vi "Plot Times.vi"(8 "reference 2":refnum<vi>, 9 "reference":refnum<vi>, 11 "Value":T1(array[cluster])) -> (0 "Positive Graph":cluster{dbl, dbl, i32[]}[](graph) caption="Waveform Graph", 3 "Negative Graph":cluster{dbl, dbl, i32[]}[](graph) caption="Waveform Graph")   [LabVIEW 2013]
doc: "Given Time Sequence Clusters, outputs vertical lines indicating relative Times\nPlots to a negative and a positive graph to allow for different scaling"
panel:
  out "Positive Graph":cluster{"X":dbl, "Y":dbl}[](graph)
  out "Negative Graph":cluster{"X":dbl, "Y":dbl}[](graph)
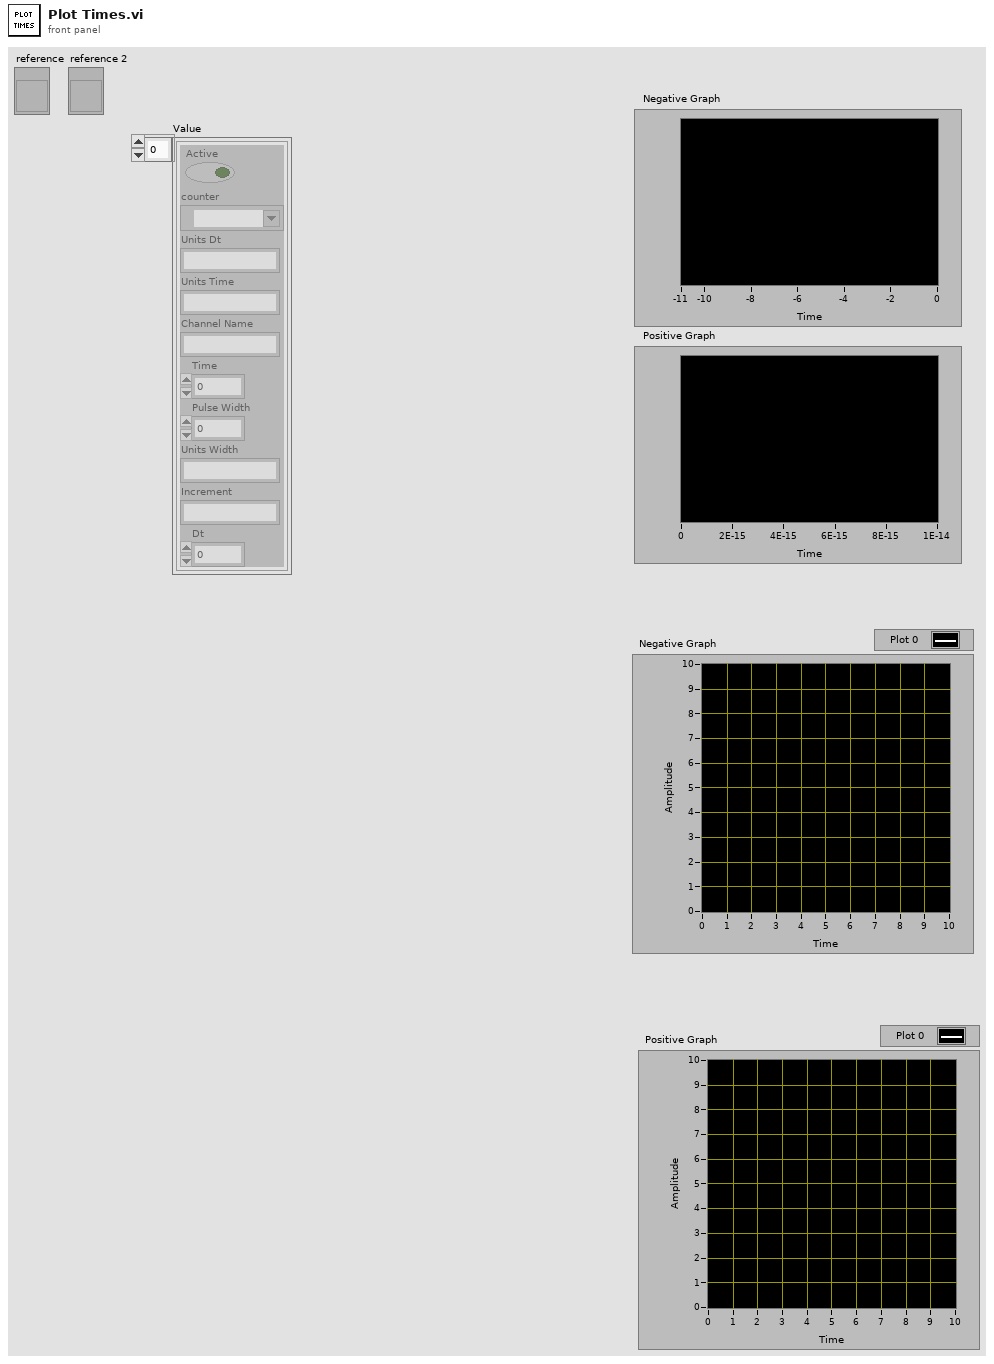
[diagram p1: front panel]
types:
  T1 = cluster{"Active":bool, "counter":tag, "Units Dt":string, "Units Time":string, "Channel Name":string, "Time":dbl, "Pulse Width":dbl, "Units Width":string, "Increment":string, "Dt":dbl}[]
  T2 = cluster{"Name":string, "Color":u32, "Style":u8, "Point Style":u8, "Name Visible":bool, "Allow Drag":bool, "Annotation Mode":u32, "Plot":i32, "Index":i32, "Position":cluster{"X":dbl, "Y":dbl}, "X Scale":u32, "Y Scale":u32, "Show Arrow":bool, "Lock Name":bool, "Plot Area":i32, "Label Offset":cluster{"X":dbl, "Y":dbl}}
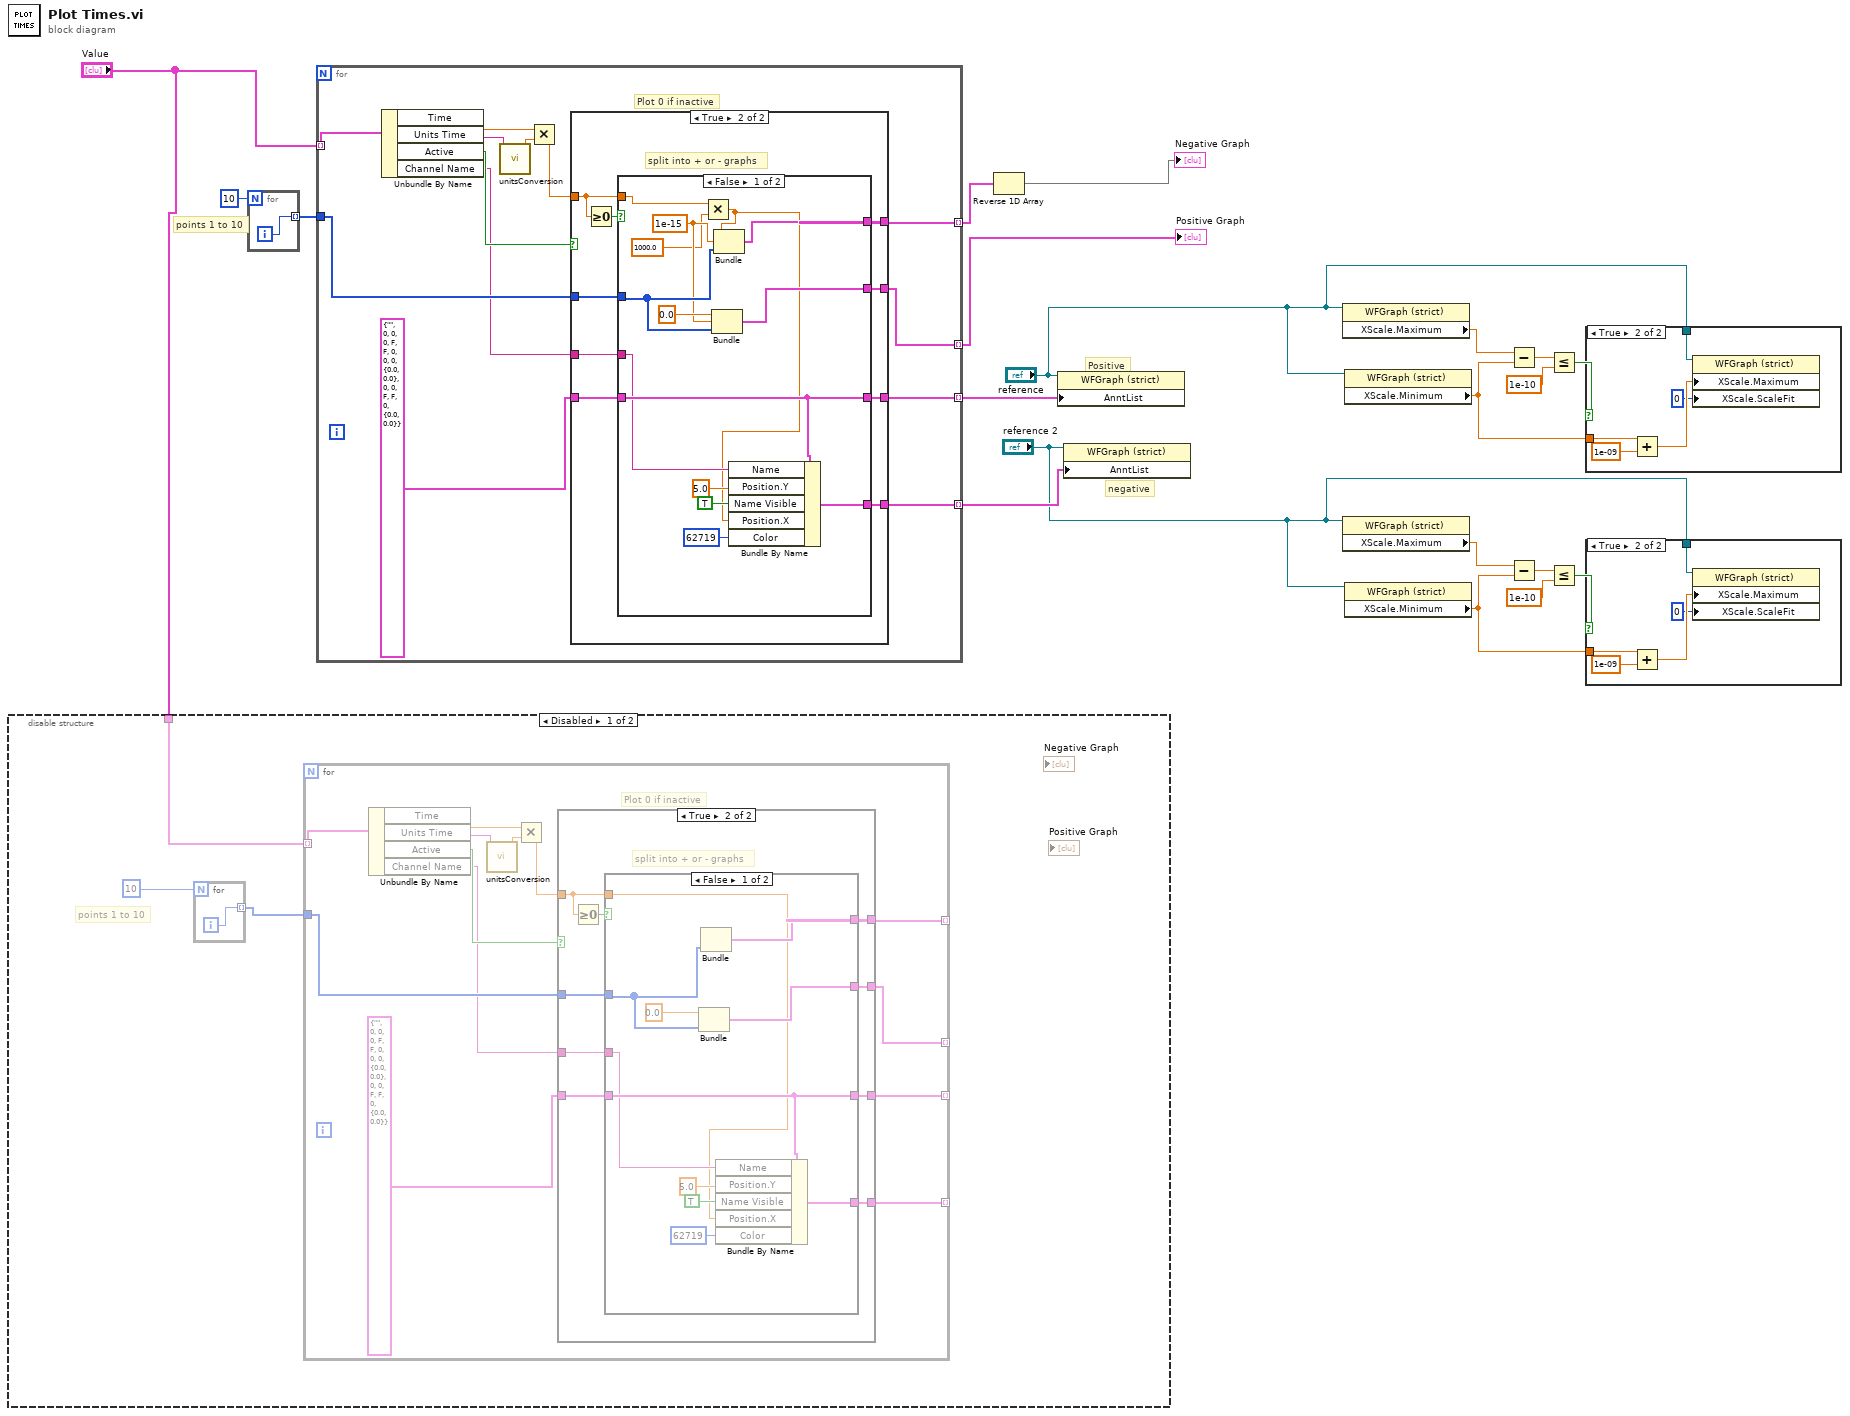
[diagram p0: block diagram]
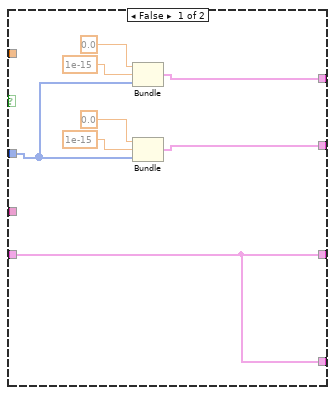
[diagram p2: hidden frame]
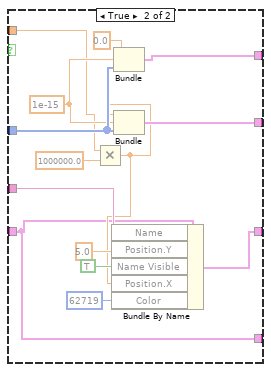
[diagram p3: hidden frame]
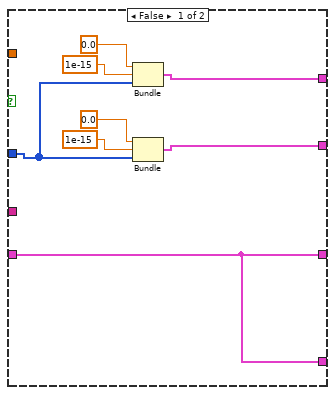
[diagram p7: hidden frame]
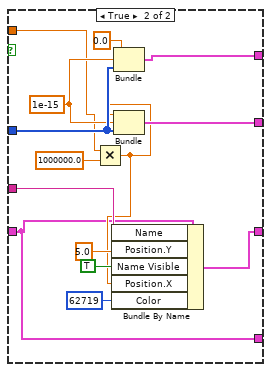
[diagram p8: hidden frame]
diagram:
  # "negative"
  # "Positive"
  # "points 1 to 10"
  n1 = disable-structure shown="Disabled" {
    disable-tunnel: "Value" -> [w23 _]
    frame Disabled {
      # "points 1 to 10"
      n2 = for {
        N: 10 -> [_]
        tunnel: [w24] -> w21 mode=indexing
        i -> [w24]
      }
      n3 = for {
        tunnel: w23 -> [w37] mode=indexing
        tunnel: w21 -> [w32]
        tunnel: [w33] -> _ mode=indexing
        tunnel: [w31] -> _ mode=indexing
        tunnel: [w27] -> _ mode=indexing
        tunnel: [w25] -> _ mode=indexing
        # "Plot 0 if inactive"
        n4 = Unbundle By Name(w37) -> ("Time"=w35:dbl, "Units Time"=w30:string, "Active"=w29:bool, "Channel Name"=w28:string)
        n5 = call "unitsConversion.vi"("Units"=w30) -> ("Numeric"=w36:dbl)  [unwired: 10 in]
        n6 = Multiply(x=w35, y=w36) -> (x*y=w34:dbl)
        n7 = case shown="True" w29 {
          tunnel: w34 -> [_ w53]
          tunnel: [w45 w52] -> w33
          tunnel: w32 -> [w39 w51]
          tunnel: [w40 w50] -> w31
          tunnel: w28 -> [_ w49]
          tunnel: T2 {"Name"="", "Color"=0, "Style"=0, "Point Style"=0, "Name Visible"=FALSE, "Allow Drag"=FALSE, "Annotation Mode"=0, "Plot"=0, "Index"=0, "Position"={"X"=0.0, "Y"=0.0}, "X Scale"=0, "Y Scale"=0, "Show Arrow"=FALSE, "Lock Name"=FALSE, "Plot Area"=0, "Label Offset"={"X"=0.0, "Y"=0.0}} -> [w38 w48]
          tunnel: [w38 w47] -> w27
          tunnel: [w38 w46] -> w25
          frame False {
            n8 = Bundle(0.0, 1e-15, w39) -> (w40:cluster{dbl, dbl, i32[]})  [unwired: 1 in]
            n9 = Bundle(0.0, 1e-15, w39) -> (w45:cluster{dbl, dbl, i32[]})  [unwired: 1 in]
          }
          frame True {
            # "split into + or - graphs"
            n10 = Greater Or Equal To 0?(x=w53) -> (x >= 0?=w54:bool)
            n11 = case shown="False" w54 {
              tunnel: w53 -> [w55 w69]
              tunnel: [w62 w79] -> w52
              tunnel: w51 -> [w63 w77]
              tunnel: [w65 w75] -> w50
              tunnel: w49 -> [w56 w74]
              tunnel: w48 -> [w58 w66]
              tunnel: [w58 w68] -> w47
              tunnel: [w57 w66] -> w46
              frame False {
                n12 = Bundle(0.0, w63) -> (w62:cluster{dbl, void, i32[]})  [unwired: 2 in]
                n13 = Bundle(w63) -> (w65:cluster{void, void, i32[]})  [unwired: 3 in]
                n14 = Bundle By Name(cluster=w58, "Name"=w56, "Position.Y"=5.0, "Name Visible"=TRUE, "Position.X"=w55, "Color"=u32 62719) -> (w57:T2)
              }
              frame True {
                w76 = 1e-15
                n15 = Multiply(x=w69, y=1000000.0) -> (x*y=w67:dbl)
                n16 = Bundle By Name(cluster=w66, "Name"=w74, "Position.Y"=5.0, "Name Visible"=TRUE, "Position.X"=w67, "Color"=u32 62719) -> (w68:T2)
                n17 = Bundle(0.0, w76, w77) -> (w75:cluster{dbl, dbl, i32[]})  [unwired: 1 in]
                n18 = Bundle(w67, w76, w77) -> (w79:cluster{dbl, dbl, i32[]})  [unwired: 1 in]
              }
            }
          }
        }
      }
    }
    frame Enabled {
    }
  }
  n19 = for {
    N: 10 -> [_]
    tunnel: [w80] -> w19 mode=indexing
    i -> [w80]
  }
  n20 = for {
    tunnel: "Value" -> [w93] mode=indexing
    tunnel: w19 -> [w88]
    tunnel: [w89] -> w18 mode=indexing
    tunnel: [w87] -> w17 mode=indexing
    tunnel: [w83] -> w15 mode=indexing
    tunnel: [w81] -> w14 mode=indexing
    # "Plot 0 if inactive"
    n21 = Unbundle By Name(w93) -> ("Time"=w91:dbl, "Units Time"=w86:string, "Active"=w85:bool, "Channel Name"=w84:string)
    n22 = call "unitsConversion.vi"("Units"=w86) -> ("Numeric"=w92:dbl)  [unwired: 10 in]
    n23 = Multiply(x=w91, y=w92) -> (x*y=w90:dbl)
    n24 = case shown="True" w85 {
      tunnel: w90 -> [_ w109]
      tunnel: [w101 w108] -> w89
      tunnel: w88 -> [w95 w107]
      tunnel: [w96 w106] -> w87
      tunnel: w84 -> [_ w105]
      tunnel: T2 {"Name"="", "Color"=0, "Style"=0, "Point Style"=0, "Name Visible"=FALSE, "Allow Drag"=FALSE, "Annotation Mode"=0, "Plot"=0, "Index"=0, "Position"={"X"=0.0, "Y"=0.0}, "X Scale"=0, "Y Scale"=0, "Show Arrow"=FALSE, "Lock Name"=FALSE, "Plot Area"=0, "Label Offset"={"X"=0.0, "Y"=0.0}} -> [w94 w104]
      tunnel: [w94 w103] -> w83
      tunnel: [w94 w102] -> w81
      frame False {
        n25 = Bundle(0.0, 1e-15, w95) -> (w96:cluster{dbl, dbl, i32[]})  [unwired: 1 in]
        n26 = Bundle(0.0, 1e-15, w95) -> (w101:cluster{dbl, dbl, i32[]})  [unwired: 1 in]
      }
      frame True {
        # "split into + or - graphs"
        n27 = Greater Or Equal To 0?(x=w109) -> (x >= 0?=w110:bool)
        n28 = case shown="False" w110 {
          tunnel: w109 -> [w118 w128]
          tunnel: [w120 w138] -> w108
          tunnel: w107 -> [w122 w136]
          tunnel: [w124 w134] -> w106
          tunnel: w105 -> [w112 w133]
          tunnel: w104 -> [w114 w125]
          tunnel: [w114 w127] -> w103
          tunnel: [w113 w125] -> w102
          frame False {
            w121 = 1e-15
            n29 = Multiply(x=w118, y=1000.0) -> (x*y=w111:dbl)
            n30 = Bundle(0.0, w121, w122) -> (w120:cluster{dbl, dbl, i32[]})  [unwired: 1 in]
            n31 = Bundle(w111, w121, w122) -> (w124:cluster{dbl, dbl, i32[]})  [unwired: 1 in]
            n32 = Bundle By Name(cluster=w114, "Name"=w112, "Position.Y"=5.0, "Name Visible"=TRUE, "Position.X"=w111, "Color"=u32 62719) -> (w113:T2)
          }
          frame True {
            w135 = 1e-15
            n33 = Multiply(x=w128, y=1000000.0) -> (x*y=w126:dbl)
            n34 = Bundle By Name(cluster=w125, "Name"=w133, "Position.Y"=5.0, "Name Visible"=TRUE, "Position.X"=w126, "Color"=u32 62719) -> (w127:T2)
            n35 = Bundle(0.0, w135, w136) -> (w134:cluster{dbl, dbl, i32[]})  [unwired: 1 in]
            n36 = Bundle(w126, w135, w136) -> (w138:cluster{dbl, dbl, i32[]})  [unwired: 1 in]
          }
        }
      }
    }
  }
  "Positive Graph" <- w18
  n37 = Reverse 1D Array(array=w17) -> (reversed array=→"Negative Graph":cluster{dbl, dbl, i32[]}[])
  n38 = property on="Property Node" class="WFGraph (strict)"(reference="reference", "AnntList"=w15) -> ()  [unwired: 1 in, 2 out]
  n39 = property on="Property Node" class="WFGraph (strict)"(reference="reference 2", "AnntList"=w14) -> ()  [unwired: 1 in, 2 out]
  n40 = property on="Property Node" class="WFGraph (strict)"(reference="reference") -> ("XScale.Maximum"=w13:dbl)  [unwired: 1 in, 2 out]
  n41 = property on="Property Node" class="WFGraph (strict)"(reference="reference 2") -> ("XScale.Maximum"=w8:dbl)  [unwired: 1 in, 2 out]
  n42 = property on="Property Node" class="WFGraph (strict)"(reference="reference") -> ("XScale.Minimum"=w9:dbl)  [unwired: 1 in, 2 out]
  n43 = property on="Property Node" class="WFGraph (strict)"(reference="reference 2") -> ("XScale.Minimum"=w4:dbl)  [unwired: 1 in, 2 out]
  n44 = Subtract(x=w13, y=w9) -> (x-y=w12:dbl)
  n45 = Subtract(x=w8, y=w4) -> (x-y=w7:dbl)
  n46 = Less Or Equal?(x=w12, y=1e-10) -> (x <= y?=w10:bool)
  n47 = Less Or Equal?(x=w7, y=1e-10) -> (x <= y?=w5:bool)
  n48 = case shown="True" w10 {
    tunnel: w9 -> [_ w143]
    tunnel: "reference" -> [_ w140]
    frame False {
    }
    frame True {
      n49 = Add(x=w143, y=1e-09) -> (x+y=w141:dbl)
      n50 = property on="Property Node" class="WFGraph (strict)"(reference=w140, "XScale.Maximum"=w141, "XScale.ScaleFit"=u8 0 ("X Scale.Scale Fit")) -> ()  [unwired: 1 in, 2 out]
    }
  }
  n51 = case shown="True" w5 {
    tunnel: w4 -> [_ w148]
    tunnel: "reference 2" -> [_ w145]
    frame False {
    }
    frame True {
      n52 = Add(x=w148, y=1e-09) -> (x+y=w146:dbl)
      n53 = property on="Property Node" class="WFGraph (strict)"(reference=w145, "XScale.Maximum"=w146, "XScale.ScaleFit"=u8 0 ("X Scale.Scale Fit")) -> ()  [unwired: 1 in, 2 out]
    }
  }
